vi "Calibration_Quadruple_Save.vi"(0 "Data":T2={"system"={"info"={"menuSelect"=0, "version"=0, "serial"="", "captureActive"=FALSE, "captureBegin"=FALSE, "emptyAndRefill"=FALSE}, "userInfo"={"operatorName"="", "date"=timestamp(2713993200 s since 1904-01-01)}, "camera"={"exposureTime"=0, "aperture"=enum."Item 0", "framerate"=0, "framerateMax"=0, "legacyAttributes"=FALSE}}, "connections"={"arduino"={"connection"="", "status"=FALSE, "openState"=FALSE, "emptyStart"=0}, "pump"={"connection"="", "status"=FALSE, "command"="", "dispenseSpeed"=0, "flushSize"=0}, "camera"={"cam1"={"connection"="", "status"=FALSE}, "cam2"={"connection"="", "status"=FALSE}}}, "queue"={"process"={"cam1"=refnum, "cam2"=refnum, "queueSize"=0}, "save"={"cam1"=refnum, "cam2"=refnum, "queueSize"=0}, "overloadThreshold"=0}, "imageProcess"={"cam1"={"preAllocation"={"image"=refnum, "originalDisplay"=refnum, "originalRgb"=refnum, "binary"=refnum, "save"=refnum, "calibrationFull"=refnum, "calibrationDetect"=refnum}, "calibration"={"pathFull"=path "", "pathDetect"=path "", "ROI"={"Left"=0, "Top"=0, "Right"=0, "Bottom"=0, "Rotation"=0.0}}}, "cam2"={"preAllocation"={"image"=refnum, "originalDisplay"=refnum, "originalRgb"=refnum, "binary"=refnum, "save"=refnum, "calibrationFull"=refnum, "calibrationDetect"=refnum}, "calibration"={"pathFull"=path "", "pathDetect"=path "", "ROI"={"Left"=0, "Top"=0, "Right"=0, "Bottom"=0, "Rotation"=0.0}}}, "process"={"planeExtract"=refnum, "planeSubtract"=refnum, "cropMask"=refnum}, "detection"={"sampleTimeout"=200, "sizeThreshold"=500, "detectionRegionPct"=0.0}}, "sampleData"={"sampleId"="", "projectId"="", "voucherID"="", "speciesName"="", "collectionDate"=timestamp(2713993200 s since 1904-01-01), "sampleStation"="", "location"="", "lat"=0.0, "lon"=0.0, "determiner"="", "sex"="", "otherNotes"=""}, "Session In"=""} {"sampleData"."collectionDate" format="%<%Y-%m-%d>T"; "imageProcess"."detection"."sizeThreshold" min=1; "imageProcess"."cam2"."calibration"."ROI"."Rotation" format="%.2f"; "imageProcess"."cam2"."calibration"."ROI"."Left" scale=0.0..1024.0; "imageProcess"."cam2"."calibration"."ROI"."Right" scale=0.0..1024.0; "imageProcess"."cam1"."calibration"."ROI"."Rotation" format="%.2f"; "imageProcess"."cam1"."calibration"."ROI"."Left" scale=0.0..1024.0; "imageProcess"."cam1"."calibration"."ROI"."Right" scale=0.0..1024.0; "queue"."overloadThreshold" min=1; "queue"."save"."queueSize" min=1; "queue"."process"."queueSize" min=1; "connections"."pump"."flushSize" min=1; "connections"."pump"."dispenseSpeed" min=1; "system"."camera"."framerateMax" min=1; "system"."userInfo"."date" format="%<%Y-%m-%dT%H:%M:%S+%z>T"; "system"."info"."version" items=["Standard", "XL"]; "system"."info"."menuSelect" items=["Session Data", "Extended Setup", "Buffer", "Camera", "Dispenser", "Stats", "Connections"]}, 5 "Img1":T1, 7 "Img2":T1, 9 "Path1":string, 11 "Path2":string) -> (4 "Cal1":path, 6 "Cal2":path, 10 "Img1 out":T1, 15 "Img2 out":T1)   [LabVIEW 2022 SP3]
uses:
  <vilib>/vision/Image Controls.llb/IMAQ Image.ctl
  <vilib>/userdefined/High Color/IMAQdx.ctl
  controls/Data.ctl
panel:
  out "error out 4":errorcluster
  out "error out 3":errorcluster
  out "error out 2":errorcluster
  out "error out":errorcluster
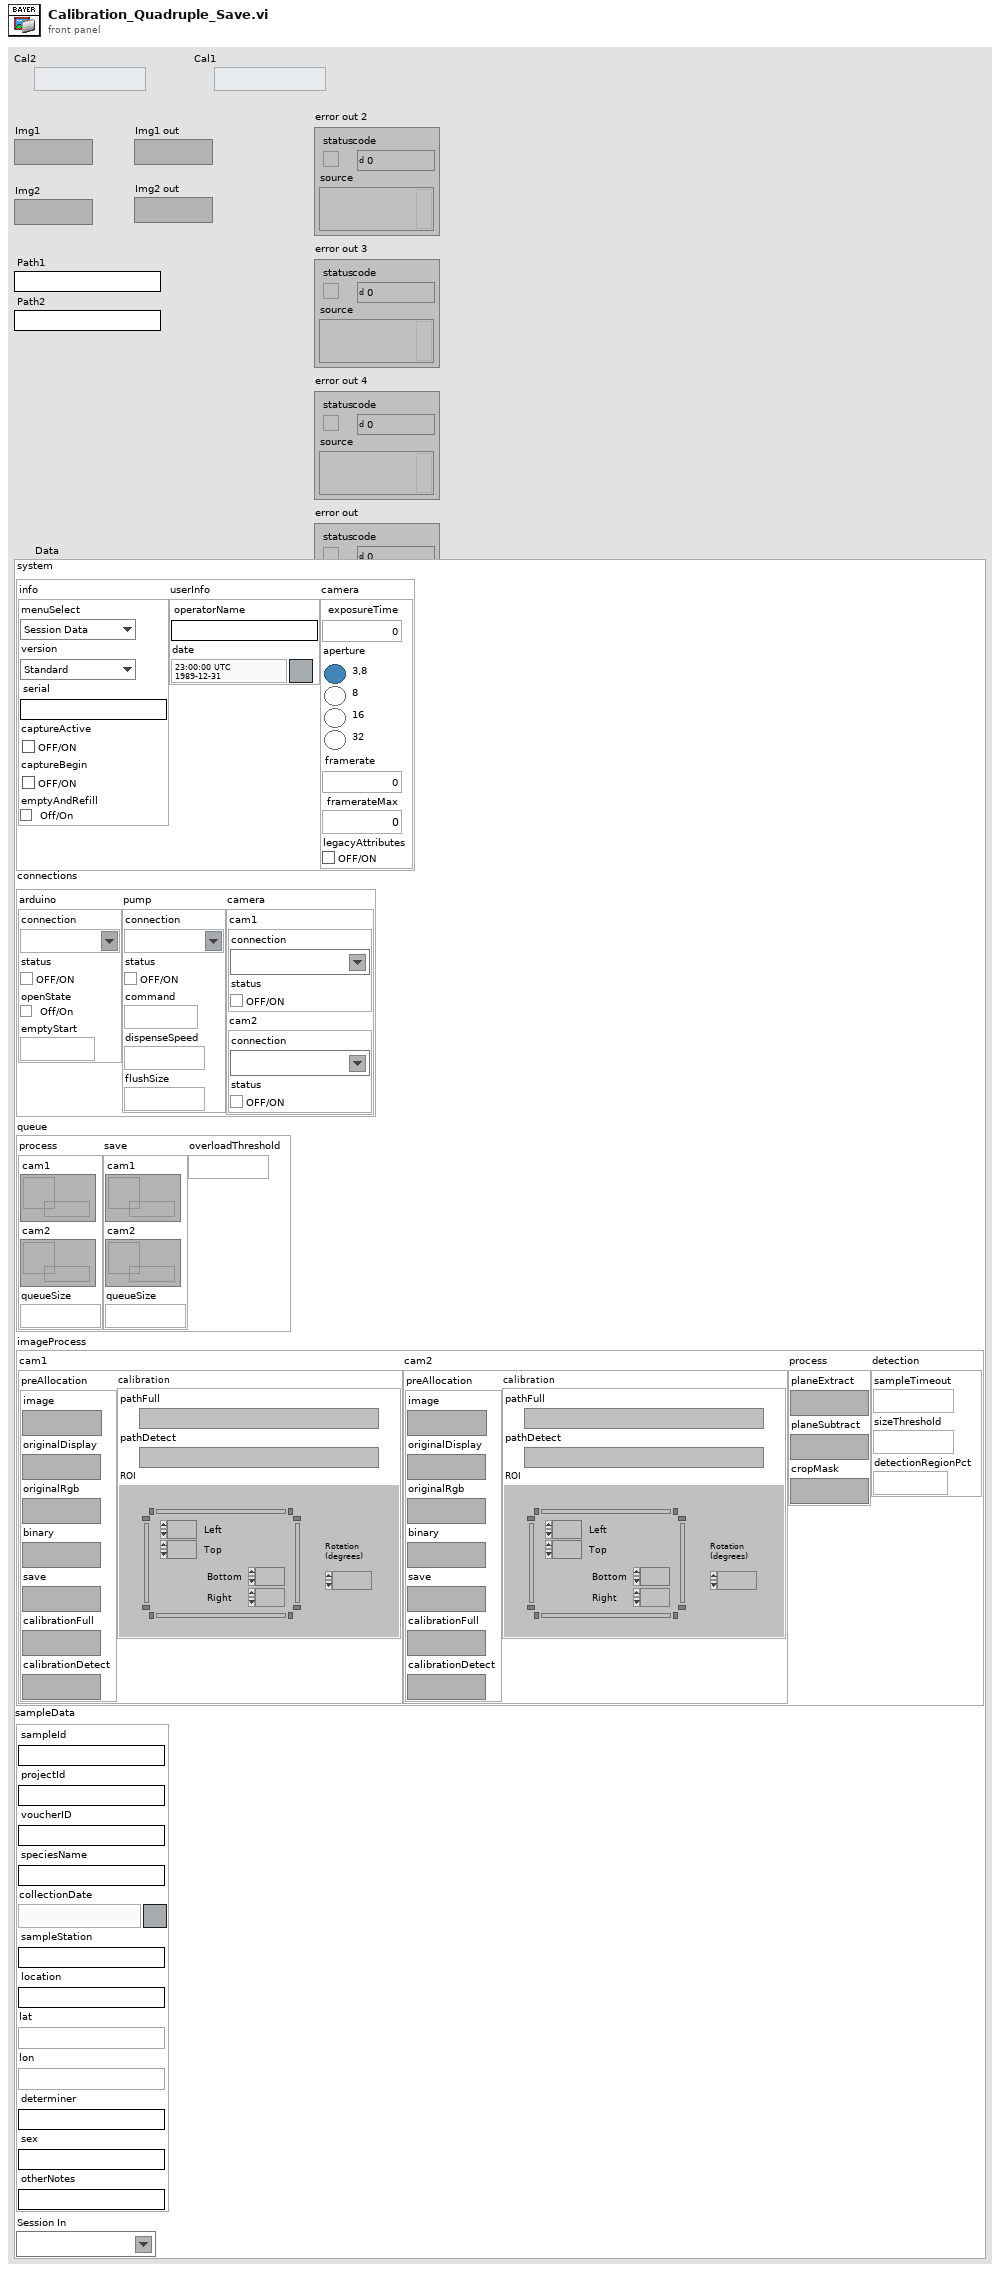
[diagram p1: front panel]
types:
  T1 = typedef "IMAQ Image.ctl" = refnum<image>
  T2 = typedef "Data.ctl" = cluster{"system":cluster{"info":cluster{"menuSelect":u16, "version":u16, "serial":string, "captureActive":bool, "captureBegin":bool, "emptyAndRefill":bool}, "userInfo":cluster{"operatorName":string, "date":timestamp}, "camera":cluster{"exposureTime":i32, "aperture":enum32{"Item 0", "Item 1", "Item 2", "Item 3"}, "framerate":i32, "framerateMax":i32, "legacyAttributes":bool}}, "connections":cluster{"arduino":cluster{"connection":refnum<visa-resource-name>, "status":bool, "openState":bool, "emptyStart":u32}, "pump":cluster{"connection":refnum<visa-resource-name>, "status":bool, "command":string, "dispenseSpeed":i32, "flushSize":i32}, "camera":cluster{"cam1":cluster{"connection":T3, "status":bool}, "cam2":cluster{"connection":T3, "status":bool}}}, "queue":cluster{"process":cluster{"cam1":refnum<queue>, "cam2":refnum<queue>, "queueSize":i32}, "save":cluster{"cam1":refnum<queue>, "cam2":refnum<queue>, "queueSize":i32}, "overloadThreshold":i32}, "imageProcess":cluster{"cam1":cluster{"preAllocation":cluster{"image":T1, "originalDisplay":T1, "originalRgb":T1, "binary":T1, "save":T1, "calibrationFull":T1, "calibrationDetect":T1}, "calibration":cluster{"pathFull":path, "pathDetect":path, "ROI":T4}}, "cam2":cluster{"preAllocation":cluster{"image":T1, "originalDisplay":T1, "originalRgb":T1, "binary":T1, "save":T1, "calibrationFull":T1, "calibrationDetect":T1}, "calibration":cluster{"pathFull":path, "pathDetect":path, "ROI":T4}}, "process":cluster{"planeExtract":T1, "planeSubtract":T1, "cropMask":T1}, "detection":cluster{"sampleTimeout":i32, "sizeThreshold":i32, "detectionRegionPct":dbl}}, "sampleData":cluster{"sampleId":string, "projectId":string, "voucherID":string, "speciesName":string, "collectionDate":timestamp, "sampleStation":string, "location":string, "lat":dbl, "lon":dbl, "determiner":string, "sex":string, "otherNotes":string}, "Session In":T3}
  T3 = typedef "IMAQdx.ctl" = refnum<k21>
  T4 = typedef "IMAQ Rectangle" = cluster{"Left":i32, "Top":i32, "Right":i32, "Bottom":i32, "Rotation":dbl}
  T5 = cluster{"Pattern":i32, "Algorithm":i32, "Red Gain":dbl, "Green Gain":dbl, "Blue Gain":dbl}
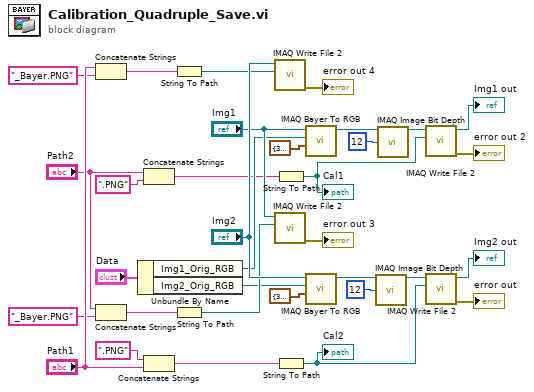
[diagram p0: block diagram]
diagram:
  n1 = Concatenate Strings("Path1", "_Bayer.PNG" ("string")) -> (w30:string)
  n2 = Concatenate Strings("Path2", "_Bayer.PNG" ("string")) -> (w21:string)
  n3 = Unbundle By Name("Data") -> ("Img1_Orig_RGB"=w18:T1, "Img2_Orig_RGB"=w20:T1)
  n4 = Concatenate Strings("Path2", ".PNG" ("string")) -> (w15:string)
  n5 = Concatenate Strings(".PNG" ("string"), "Path1") -> (w17:string)
  n6 = String To Path(string=w30) -> (path=w32:path)
  n7 = String To Path(string=w21) -> (path=w26:path)
  n8 = call-poly "IMAQ Write File 2"("File Path"=w32, "Image"="Img2") -> ("error out"=→"error out 4":errorcluster)  [unwired: 8 in, 1 out]
  n9 = call-poly "IMAQ Write File 2"("File Path"=w26, "Image"="Img1") -> ("error out"=→"error out 3":errorcluster)  [unwired: 8 in, 1 out]
  n10 = String To Path(string=w15) -> (path=w10:path)
  "Cal1" <- w10
  n11 = String To Path(string=w17) -> (path=w7:path)
  "Cal2" <- w7
  n12 = call "IMAQ Bayer To RGB"("Bayer Parameters"=T5 {"Pattern"=3, "Algorithm"=0, "Red Gain"=1.0, "Green Gain"=1.0, "Blue Gain"=1.0}, "Image Dst"=w18, "Image Src"="Img1") -> ("Image Dst Out"=w2:T1)  [unwired: 7 in, 1 out]
  n13 = call "IMAQ Bayer To RGB"("Bayer Parameters"=T5 {"Pattern"=3, "Algorithm"=0, "Red Gain"=1.0, "Green Gain"=1.0, "Blue Gain"=1.0}, "Image Dst"=w20, "Image Src"="Img2") -> ("Image Dst Out"=w5:T1)  [unwired: 7 in, 1 out]
  n14 = call "IMAQ Image Bit Depth"("Image"=w5, "Bit Depth (0)"=u32 12) -> ("Image Out"=w4:T1)  [unwired: 11 in, 2 out]
  n15 = call "IMAQ Image Bit Depth"("Image"=w2, "Bit Depth (0)"=u32 12) -> ("Image Out"=w1:T1)  [unwired: 11 in, 2 out]
  n16 = call-poly "IMAQ Write File 2"("File Path"=w10, "Image"=w1) -> ("error out"=→"error out 2":errorcluster, "Image Out (duplicate)"=→"Img1 out":T1)  [unwired: 8 in]
  n17 = call-poly "IMAQ Write File 2"("File Path"=w7, "Image"=w4) -> ("error out"=→"error out":errorcluster, "Image Out (duplicate)"=→"Img2 out":T1)  [unwired: 8 in]
